vi "New Terminal Reference Binding.vi"(10 "Ctl Refnum":refnum<vi>) -> (0 "error out":errorcluster, 3 "TerminalReference out":refnum<class "TerminalReference.lvclass">)   [LabVIEW 2015, in "Mediator.lvlib" / "TerminalReference.lvclass"]
uses:
  TerminalReference.lvclass
  TerminalReference.lvclass/TerminalReference.ctl
panel:
  # "Immediately DEPRECATED.\nUse TerminalBinding.lvclass--It's\nway faster and does the same thing"
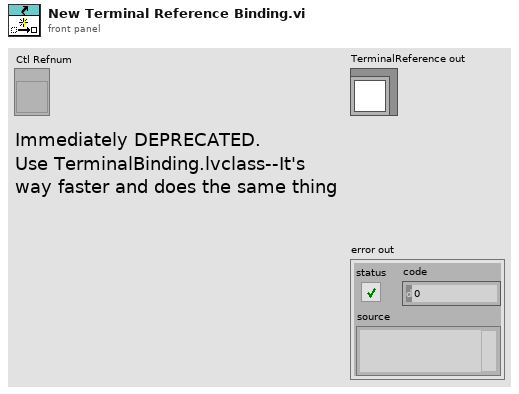
[diagram p1: front panel]
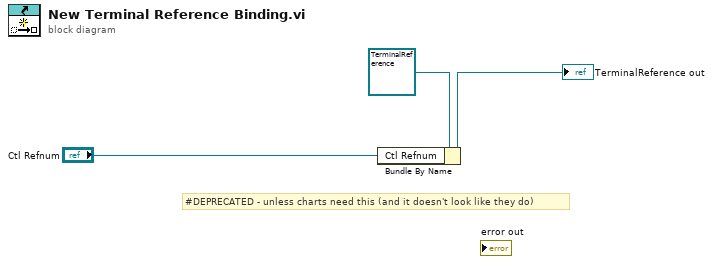
[diagram p0: block diagram]
diagram:
  # "#DEPRECATED - unless charts need this (and it doesn't look like they do)"
  n1 = Bundle By Name(cluster=refnum<class "TerminalReference.lvclass"> refnum ("TerminalReference in"), "Ctl Refnum"="Ctl Refnum") -> (→"TerminalReference out":refnum<class "TerminalReference.lvclass">)
